vi "WD Polling (subVI).vi"(3 "Timer Initialize (ms)":u32, 4 "Timeout (ms)":u32, 5 "Whack":bool, 6 "Arm":bool) -> (0 "Expired":bool)   [LabVIEW 2015]
doc: "This subVI supports a watchdog timer host VI. When the Arm control is set, this VI determines whether a timeout has occured before the Whack control has been last set. If a timeout occurs, the Expired indicator is set and held until the Arm control is reset.\n\nThe Timer Initialize control is used to measure the first value of the clock in ms when the host is initialized."
panel:
  # "This subVI supports a watchdog timer host VI. When the Arm control is set, this VI determines whether a timeout has occured before the Whack control has been last set.  If a timeout occurs, the Expired indicator is set and held until the Arm control is reset.\n\nThe Timer Initialize control is used to measure the first value of the clock in ms when the host is initialized."
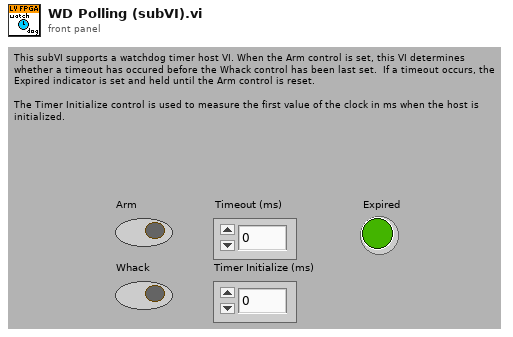
[diagram p1: front panel]
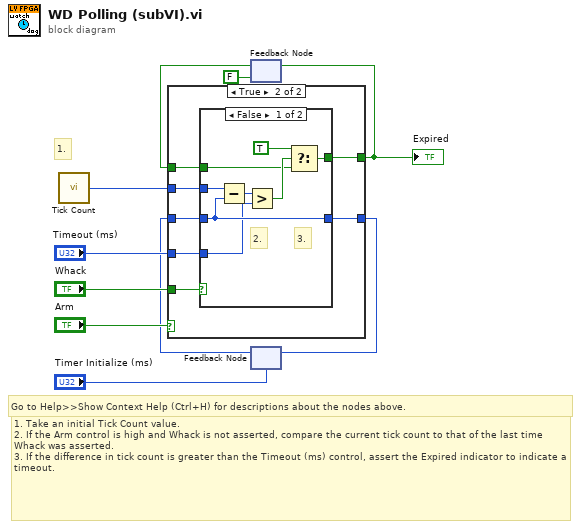
[diagram p0: block diagram]
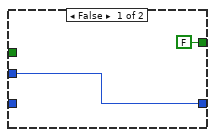
[diagram p2: hidden frame]
diagram:
  # "1."
  # "Go to Help>>Show Context Help (Ctrl+H) for descriptions about the nodes above."
  # "1. Take an initial Tick Count value.\n2. If the Arm control is high and Whack is not asserted, compare the current tick count to that of the last time Whack was asserted.\n3. If the difference in tick count is greater than the Timeout (ms) control, assert the Expired indicator to indicate a timeout."
  n1 = call "Tick Count"() -> ("Tick Count(mSec)"=w1:u32)
  n2 = feedback #1(FALSE ("t")) -> (w7:bool)
  n3 = feedback #2("Timer Initialize (ms)") -> (w3:u32)
  n4 = case shown="True" "Arm" {
    tunnel: w1 -> [w12 w17]
    tunnel: "Whack" -> [_ w19]
    tunnel: [w12 w18] -> w4
    tunnel: [FALSE w16] -> w8
    tunnel: w7 -> [_ w15]
    tunnel: w3 -> [_ w14]
    tunnel: "Timeout (ms)" -> [_ w13]
    frame False {
    }
    frame True {
      n5 = case shown="False" w19 {
        tunnel: [w21 w29] -> w18
        tunnel: w17 -> [w27 w29]
        tunnel: [w22 w28] -> w16
        tunnel: w15 -> [w23 w28]
        tunnel: w14 -> [w21 _]
        tunnel: w13 -> [w20 _]
        frame False {
          # "3."
          # "2."
          n6 = Subtract(x=w27, y=w21) -> (x-y=w26:u32)
          n7 = Greater?(x=w26, y=w20) -> (0:w24:bool)
          n8 = Select(t=TRUE, s=w24, f=w23) -> (s? t:f=w22:bool)
        }
        frame True {
        }
      }
    }
  }
  "Expired" <- w8
  n9 = feedback-in #1(w8) -> ()
  n10 = feedback-in #2(w4) -> ()
